vi "Add Nested Enq.vi"(7 "Ident":string, 10 "Nested Actor's Enqueuer":refnum<class "Message Enqueuer.lvclass">, 11 "Interactor in":refnum<class "Interactor.lvclass">) -> (3 "Interactor out":refnum<class "Interactor.lvclass">)   [LabVIEW 2020, in "Interactor.lvlib" / "Interactor.lvclass"]
uses:
  Interactor.lvclass
  Interactor.lvclass/Interactor.ctl
  <vilib>/ActorFramework/Message Enqueuer/Message Enqueuer.lvclass
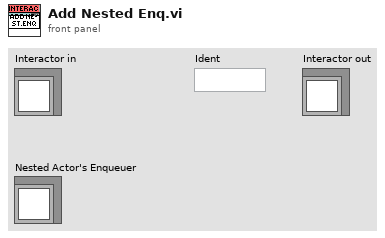
[diagram p1: front panel]
types:
  T1 = map{string, refnum<class "Message Enqueuer.lvclass">}
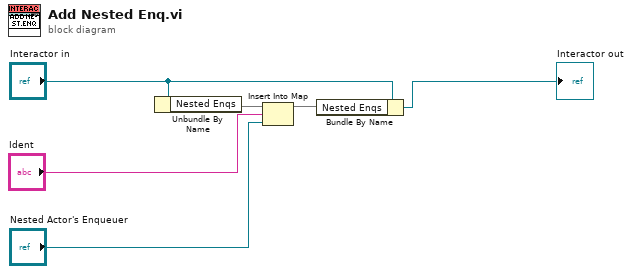
[diagram p0: block diagram]
diagram:
  n1 = Unbundle By Name("Interactor in") -> ("Nested Enqs"=w6:T1)
  n2 = Insert Into Map(map in=w6, key="Ident", value="Nested Actor's Enqueuer") -> (map out=w3:T1)  [unwired: 2 out]
  n3 = Bundle By Name(cluster="Interactor in", "Nested Enqs"=w3) -> (→"Interactor out":refnum<class "Interactor.lvclass">)
